vi "PPG_ABCGUI.contents.vi"   [LabVIEW 2014, in "PPG_ABCGUI.lvlib"]
doc: "loads all VIs into memory - required for building an application"
uses:
  PPG_ABCGUI.lvlib
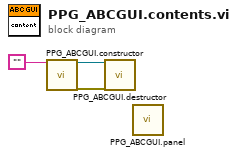
[diagram p0: block diagram]
diagram:
  n1 = call "PPG_ABCGUI.constructor.vi"("name"="") -> ("i ref out"=w3:refnum<vi>, "error out"=w2:errorcluster)  [unwired: 16 in, 1 out]
  n2 = call "PPG_ABCGUI.destructor.vi"("i ref in"=w3, "error in (no error)"=w2) -> ()  [unwired: 17 in, 1 out]
  n3 = call "PPG_ABCGUI.panel.vi"() -> ()  [unwired: 1 in]
